vi "Launcher.vi"() -> ()   [LabVIEW 2020]
uses:
  <vilib>/ActorFramework/Message Enqueuer/Message Enqueuer.lvclass
  <vilib>/ActorFramework/Message Enqueuer/Message Enqueuer.lvclass/Message Enqueuer.ctl
  GUI_Graph/GUI_Graph.lvclass
  C:/Program Files/National Instruments/LabVIEW 2020/vi.lib/ActorFramework/Actor/Actor.lvclass
  Contador_binario/Contador_binario/Contador_binario.lvclass
  <vilib>/ActorFramework/Message Enqueuer/Enqueue.vi
  <vilib>/ActorFramework/Stop Msg/Stop Msg.lvclass
  C:/Program Files/National Instruments/LabVIEW 2020/vi.lib/ActorFramework/Message/Message.lvclass
  <vilib>/ActorFramework/Message Priority Queue/Priority Enqueue.vi
  <vilib>/ActorFramework/Actor/Actor.lvclass
panel:
  in  "stop":bool
  in  "Detener":bool
  in  "GUI para detener":u16(ring) caption="Enum 3" items=["", "Grafica 1", "Grafica 2"]
  in  "Open":bool
  in  "Tipo de GUI":u16(ring) items=["Gráfica", "Binario"]
  # "LAUNCHER"
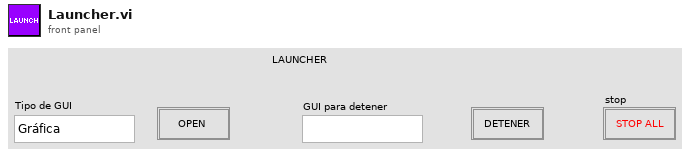
[diagram p1: front panel]
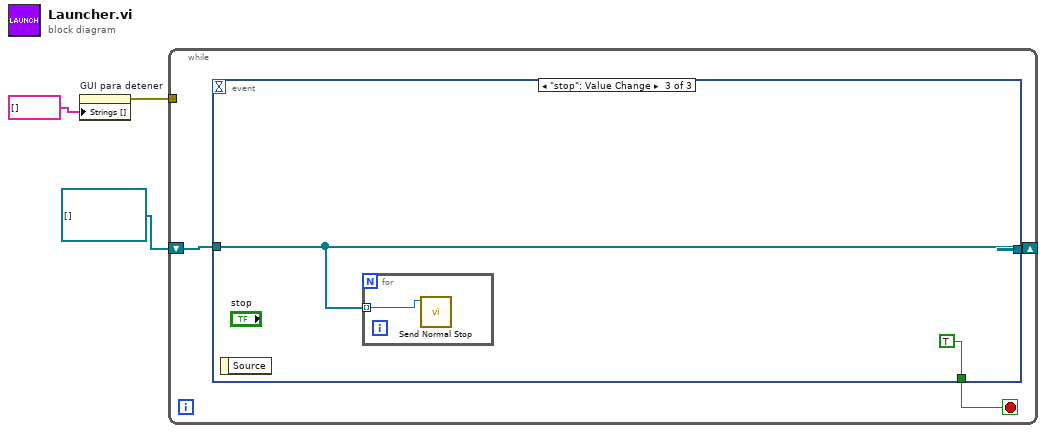
[diagram p0: block diagram]
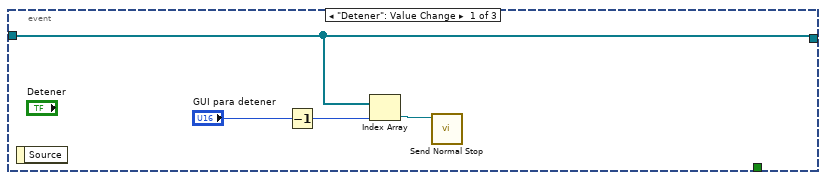
[diagram p2: hidden frame]
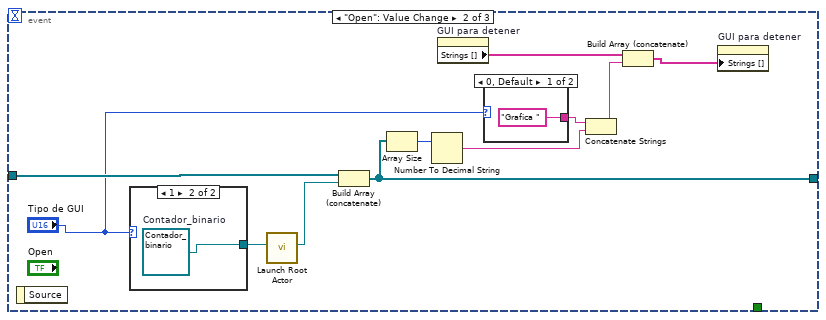
[diagram p3: hidden frame]
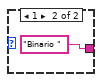
[diagram p4: hidden frame]
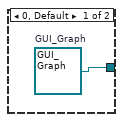
[diagram p5: hidden frame]
diagram:
  n1 = property on="GUI para detener" class="Ring (strict)"("Strings []"=string[] []) -> (error out=w1:errorcluster)  [unwired: 2 in, 1 out]
  n2 = while {
    shift-right: [w5] -> _
    shift-left: refnum<class "Message Enqueuer.lvclass">[] [] -> [w6]
    tunnel: w1 -> [_]
    stop <- w4 stop-if-true
    n3 = event shown="[2] \"stop\": Value Change" {
      selector: _ -> [_ _ _]
      dyn-events: _ -> [_ _ _]
      timeout: _ -> [_ _ _]
      tunnel: w6 -> [w9 w19 w26]
      tunnel: [w9 w17 w26] -> w5
      tunnel: [_ _ TRUE] -> w4
      event "Detener": Value Change {
        n4 = event-data() -> ()  [unwired: 1 in, 1 out]
        n5 = Decrement(x="GUI para detener") -> (x-1=w8:u16)
        n6 = Index Array(array=w9, index=w8) -> (element=w7:refnum<class "Message Enqueuer.lvclass">)
        n7 = call <vilib>:"Send Normal Stop.vi"("Message Enqueuer"=w7) -> ()  [unwired: 10 in, 1 out]
      }
      event "Open": Value Change {
        n8 = event-data() -> ()  [unwired: 1 in, 1 out]
        n9 = case shown="1" "Tipo de GUI" {
          tunnel: [w24 w25] -> w21
          frame 0, Default {
            w24 = refnum<class "GUI_Graph.lvclass"> refnum  # GUI_Graph
          }
          frame 1 {
            w25 = refnum<class "Contador_binario.lvclass"> refnum  # Contador_binario
          }
        }
        n10 = call <vilib>:"Launch Root Actor.vi"("Actor"=w21) -> ("Actor's Enqueuer"=w20:refnum<class "Message Enqueuer.lvclass">)  [unwired: 9 in, 1 out]
        n11 = Build Array (concatenate)(w19, w20) -> (w17:refnum<class "Message Enqueuer.lvclass">[])
        n12 = Array Size(array=w17) -> (size(s)=w16:i32)
        n13 = Number To Decimal String(number=w16) -> (decimal integer string=w14:string)  [unwired: 1 in]
        n14 = property on="GUI para detener" class="Ring (strict)"() -> ("Strings []"=w13:string[])  [unwired: 2 in, 2 out]
        n15 = case shown="0, Default" "Tipo de GUI" {
          tunnel: ["Grafica " ("string") "Binario " ("string")] -> w15
          frame 0, Default {
          }
          frame 1 {
          }
        }
        n16 = Concatenate Strings(w15, w14) -> (w12:string)
        n17 = Build Array (concatenate)(w13, w12) -> (w11:string[])
        n18 = property on="GUI para detener" class="Ring (strict)"("Strings []"=w11) -> ()  [unwired: 2 in, 2 out]
      }
      event "stop": Value Change {
        n19 = event-data() -> ()  [unwired: 1 in, 1 out]
        n20 = for {
          tunnel: w26 -> [w28] mode=indexing
          n21 = call <vilib>:"Send Normal Stop.vi"("Message Enqueuer"=w28) -> ()  [unwired: 10 in, 1 out]
        }
      }
    }
  }
